vi "Pre Launch Init.vi"(11 "Pressure in":refnum<class "Pressure.lvclass">) -> (0 "error out":errorcluster, 3 "Pressure out":refnum<class "Pressure.lvclass">)   [LabVIEW 2018, in "Pressure Actor.lvlib" / "Pressure.lvclass"]
doc: "(<B>Filename</B>: Actor Framework.lvlib:Actor.lvclass:Pre Launch Init.vi)\n\nDefines behavior that occurs after the Launch Nested Actor method is invoked but before the actor's Actor Core method begins running.\n\nBy default, this method does nothing. A descendant class may override it to define behavior."
uses:
  Pressure.lvclass
  <vilib>/ActorFramework/Actor/Actor.lvclass
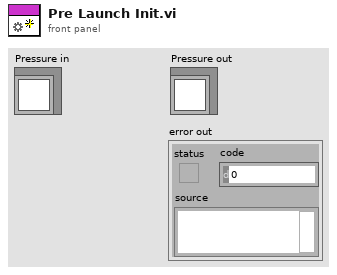
[diagram p1: front panel]
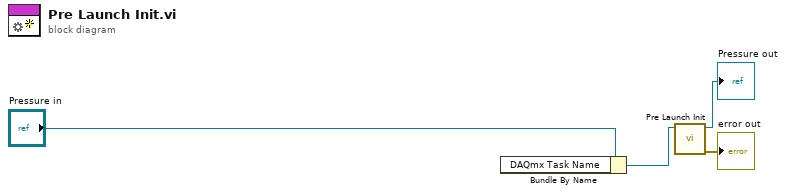
[diagram p0: block diagram]
diagram:
  n1 = Bundle By Name(cluster="Pressure in") -> (w2:refnum<class "Pressure.lvclass">)  [unwired: 1 in]
  n2 = call-parent "Pre Launch Init.vi"("Actor in"=w2) -> ("error out"=→"error out":errorcluster, "Actor out"=→"Pressure out":refnum<class "Pressure.lvclass">)  [unwired: 9 in]
